vi "ValChange.vi"(6 "Value":string, 8 "error in (no error)":errorcluster, 9 "Table CtlRef In":refnum<vi>, 10 "Cell Position":T1, 11 "DigitalCol in":refnum<class "DigitalCol.lvclass">) -> (0 "error out":errorcluster, 1 "Table CtlRef Out":refnum<vi>, 3 "DigitalCol out":refnum<class "DigitalCol.lvclass">)   [LabVIEW 2013, in "DigitalCol.lvclass"]
doc: "Similar to parent method, this VI pushes value change to disabled cells and then updates the digital cell color.\nThis VI is read-only w.r.t column data."
uses:
  DigitalCol.lvclass
  <vilib>/Utility/miscctls.llb/LVRowAndColumnTypeDef.ctl
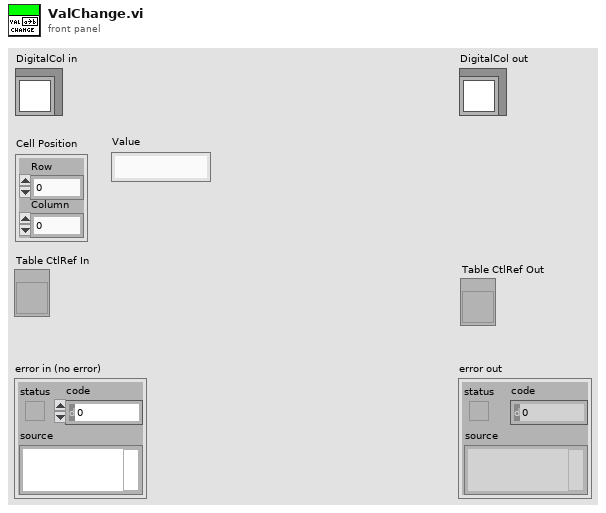
[diagram p1: front panel]
types:
  T1 = typedef "LVRowAndColumnTypeDef.ctl" = cluster{"Row":i32, "Column":i32}
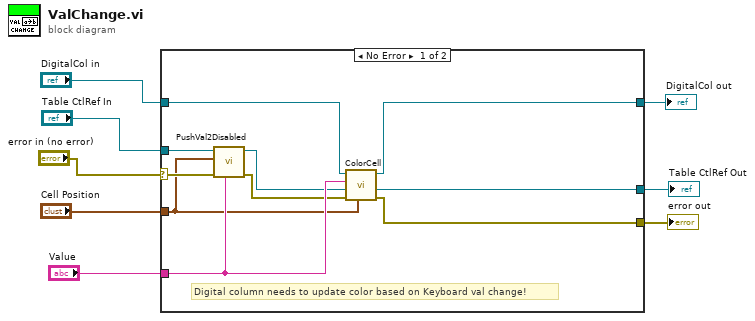
[diagram p0: block diagram]
diagram:
  n1 = case shown="No Error" "error in (no error)" {
    selector: "error in (no error)" -> [w17 w20]
    tunnel: "Table CtlRef In" -> [w18 w19]
    tunnel: [w9 w19] -> w7
    tunnel: [w16 w20] -> w6
    tunnel: "DigitalCol in" -> [w11 w21]
    tunnel: [w10 w21] -> w8
    tunnel: "Cell Position" -> [w14 _]
    tunnel: "Value" -> [w15 _]
    frame No Error {
      # "Digital column needs to update color based on Keyboard val change!"
      n2 = call "PushVal2Disabled.vi"("Value"=w15, "error in (no error)"=w17, "Cell Position"=w14, "Table CtlRef In"=w18) -> ("error out"=w13:errorcluster, "Table CtlRef Out"=w12:refnum<vi>)  [unwired: 5 in, 1 out]
      n3 = call-dynamic "ColorCell.vi"("Cell Position"=w14, "error in (no error)"=w13, "Table CtlRef In"=w12, "Value"=w15, "DigitalCol in"=w11) -> ("error out"=w16:errorcluster, "Table CtlRef Out"=w9:refnum<vi>, "DigitalCol out"=w10:refnum<class "DigitalCol.lvclass">)  [unwired: 4 in]
    }
    frame Error {
    }
  }
  "error out" <- w6
  "DigitalCol out" <- w8
  "Table CtlRef Out" <- w7
